vi "Material-SubtractLiner-Normalize.vi"(8 "error in (no error)":errorcluster, 11 "Material-RunTest in":refnum<class "Material-RunTest.lvclass">) -> (0 "error out":errorcluster, 3 "Material-RunTest out":refnum<class "Material-RunTest.lvclass">)   [LabVIEW 2013, in "Material-RunTest.lvclass"]
uses:
  Material-RunTest.lvclass
  Material-RunTest.lvclass/Material-RunTest.ctl
  <vilib>/Utility/file.llb/Read From Spreadsheet File (DBL).vi
  <vilib>/Utility/file.llb/Read From Spreadsheet File (I64).vi
  <userlib>/_OpenG.lib/array/array.llb/Search 1D Array (I32)__ogtk.vi
  <userlib>/_OpenG.lib/array/array.llb/Delete Elements from 1D Array (I32)__ogtk.vi
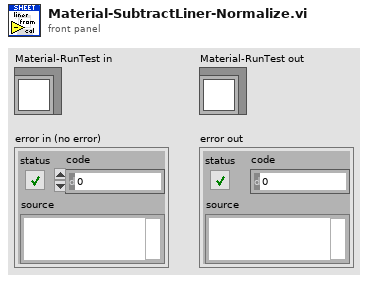
[diagram p1: front panel]
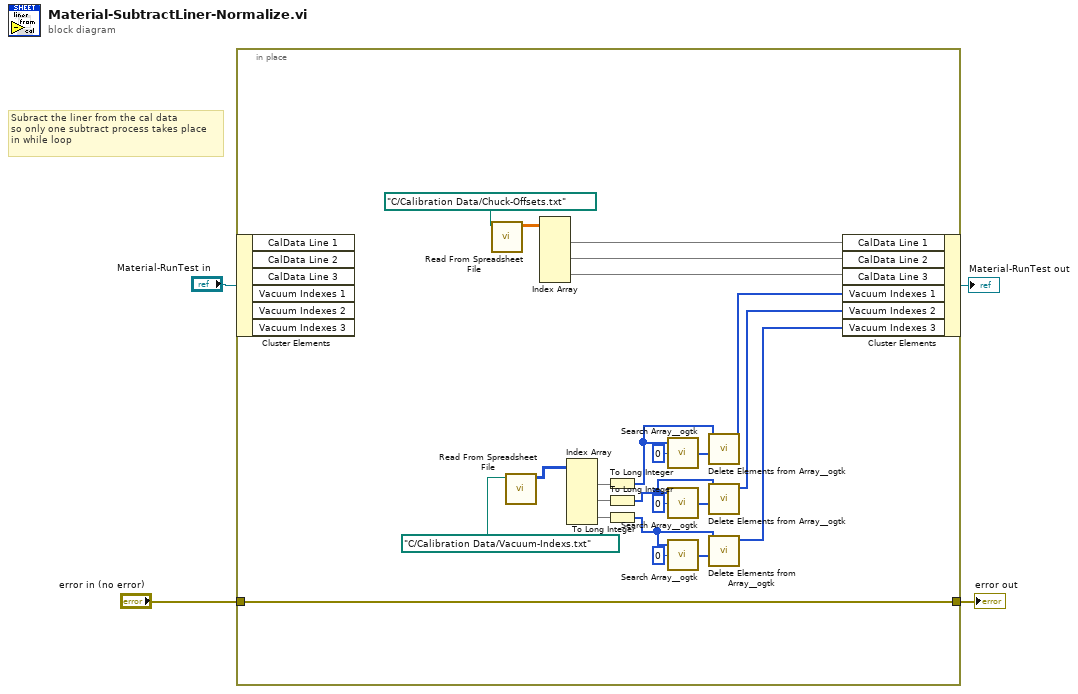
[diagram p0: block diagram]
diagram:
  # "Subract the liner from the cal data\nso only one subtract process takes place\nin while loop"
  n1 = in-place {
    in-place-border: "error in (no error)" -> [w23]
    in-place-border: [w23] -> w4
    n2 = in-place-cluster #1("Material-RunTest in") -> ()  [unwired: 6 out]
    n3 = call-poly <vilib>:"Read From Spreadsheet File.vi"("file path (dialog if empty)"=path "C:/Calibration Data/Chuck-Offsets.txt") -> ("all rows"=w27:dbl[][])  [unwired: 6 in, 4 out]
    n4 = call-poly <vilib>:"Read From Spreadsheet File.vi"("file path (dialog if empty)"=path "C:/Calibration Data/Vacuum-Indexs.txt") -> ("all rows"=w26:i64[][])  [unwired: 6 in, 4 out]
    n5 = Index Array(array=w27) -> (element #1=w7:dbl[], element #2=w6:dbl[], element #3=w5:dbl[])  [unwired: 6 in]
    n6 = Index Array(array=w26) -> (element #1=w20:i64[], element #2=w25:i64[], element #3=w24:i64[])  [unwired: 6 in]
    n7 = To Long Integer(number=w20) -> (32bit integer=w17:i32[])
    n8 = To Long Integer(number=w25) -> (32bit integer=w13:i32[])
    n9 = To Long Integer(number=w24) -> (32bit integer=w9:i32[])
    n10 = call-poly <userlib>:"Search Array__ogtk.vi"("Array"=w17, "Element Data"=0) -> ("Indices of Elements"=w18:i32[])  [unwired: 7 in]
    n11 = call-poly <userlib>:"Search Array__ogtk.vi"("Array"=w13, "Element Data"=0) -> ("Indices of Elements"=w15:i32[])  [unwired: 7 in]
    n12 = call-poly <userlib>:"Search Array__ogtk.vi"("Array"=w9, "Element Data"=0) -> ("Indices of Elements"=w10:i32[])  [unwired: 7 in]
    n13 = call-poly <userlib>:"Delete Elements from Array__ogtk.vi"("indices"=w18, "array"=w17) -> ("array w/ subset deleted"=w16:i32[])  [unwired: 8 in, 1 out]
    n14 = call-poly <userlib>:"Delete Elements from Array__ogtk.vi"("indices"=w15, "array"=w13) -> ("array w/ subset deleted"=w12:i32[])  [unwired: 8 in, 1 out]
    n15 = call-poly <userlib>:"Delete Elements from Array__ogtk.vi"("indices"=w10, "array"=w9) -> ("array w/ subset deleted"=w8:i32[])  [unwired: 8 in, 1 out]
    n16 = in-place-cluster #1("CalData Line 1"=w7, "CalData Line 2"=w6, "CalData Line 3"=w5, "Vacuum Indexes 1"=w16, "Vacuum Indexes 2"=w12, "Vacuum Indexes 3"=w8) -> (→"Material-RunTest out":refnum<class "Material-RunTest.lvclass">)
  }
  "error out" <- w4
